vi "temperature_convertor.vi"() -> ()   [LabVIEW 2020]
panel:
  out "?":dbl
  out "Temperature (Fahrenheit)":dbl(slide) scale=0.0..100.0
  in  "Temperature (Celcius)":dbl
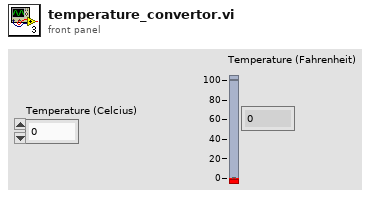
[diagram p1: front panel]
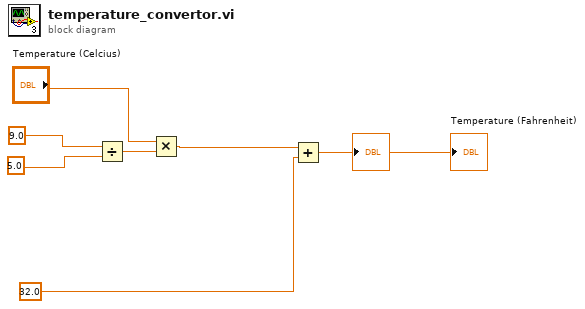
[diagram p0: block diagram]
diagram:
  n1 = Divide(x=9.0, y=5.0) -> (x/y=w4:dbl)
  n2 = Multiply(x="Temperature (Celcius)", y=w4) -> (x*y=w3:dbl)
  n3 = Add(x=w3, y=32.0) -> (x+y=→"Temperature (Fahrenheit)" →"?":dbl)
